vi "ReadTorqueWaveform.vi"(8 "error in (no error)":errorcluster, 11 "Map":T1) -> (0 "error out":errorcluster, 2 "found":bool, 3 "Torque Waveform":waveform(sgl))   [LabVIEW 2017, in "McsaUtilities.lvlib"]
uses:
  <vilib>/addons/InsightCM/Utilities/MCSA/McsaUtilities.lvlib
  <vilib>/addons/PointValueMap/controls/PointMap.ctl
  <vilib>/addons/PointValueMap/subVIs/Point_Read_variant.vi
  <vilib>/addons/PointValueMap/PointValueMap.lvlib
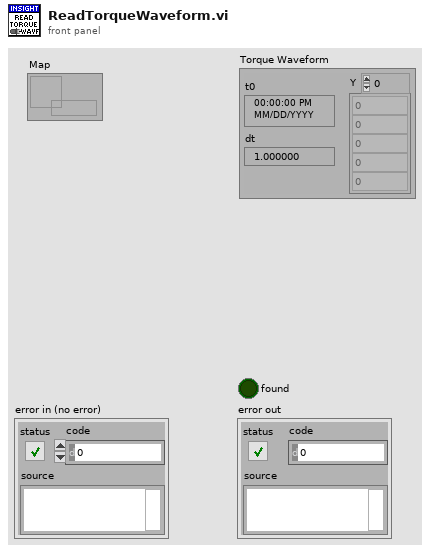
[diagram p1: front panel]
types:
  T1 = typedef "PointValueMap.lvlib/PointMap.ctl" = refnum<data-value>
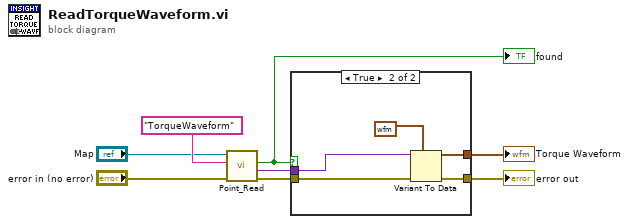
[diagram p0: block diagram]
diagram:
  n1 = call-poly <vilib>:"Point_Read.vi"("Error In"="error in (no error)", "Tag"="TorqueWaveform", "Map"="Map") -> ("Error Out"=w4:errorcluster, "Value"=w3:variant, "Found?"=w7:bool)  [unwired: 3 in, 3 out]
  "found" <- w7
  n2 = case shown="True" w7 {
    tunnel: [w9 w14] -> w2
    tunnel: w3 -> [_ w13]
    tunnel: w4 -> [w9 w12]
    tunnel: [_ w11] -> w1
    frame False {
    }
    frame True {
      n3 = Variant To Data(error in=w12, type=waveform(sgl) {"t0"=timestamp(0 s since 1904-01-01), "dt"=1.0, "Y"=[]} ("Torque Waveform"), Variant=w13) -> (data=w11:waveform(sgl), error out=w14:errorcluster)
    }
  }
  "error out" <- w2
  "Torque Waveform" <- w1
